vi "correction_data.vi"() -> ()   [LabVIEW 2020]
uses:
  CasaoManagerGeneralSpecifications.ctl
  General dimensions definition.ctl
  Point2D.ctl
  Point2Df.ctl
  WavefrontCorrector.lvclass
  Camera.lvclass
  CorrectionDataManager.lvclass
  Image.lvclass
  HasoEngine.lvclass
  InteractionMatrixAcquisitionParameters.ctl
  HasoSlopes.lvclass
  Data alignment enum.ctl
  InteractionMatrixToCommandMatrixParameters.ctl
panel:
  out "Camera Image (2N)":u32[][](graph)
  in  "Start Acq":bool
  out "Camera Image (2N+1)":u32[][](graph)
  in  "number of images to sum":u32=1
  in  "Exposure time (us)":i32=1000
  out "# of valid actuators":u32
  out "Singular values":dbl[](graph)
  in  "Correction data file name":string="Data\\data_correction_manager_example.aomi"
  in  "WavefrontCorrector Configuration file path":path
  out "error out":errorcluster
  out "Informations extracted \nfrom configuration files":T1 caption="Informations extracted from configuration files"
  in  "Haso configuration file path":path
  # "This example is Hardware-dependant, \nplease use your own Haso and corrector configuration file and acquisition system"
  # "Acquisition parameters"
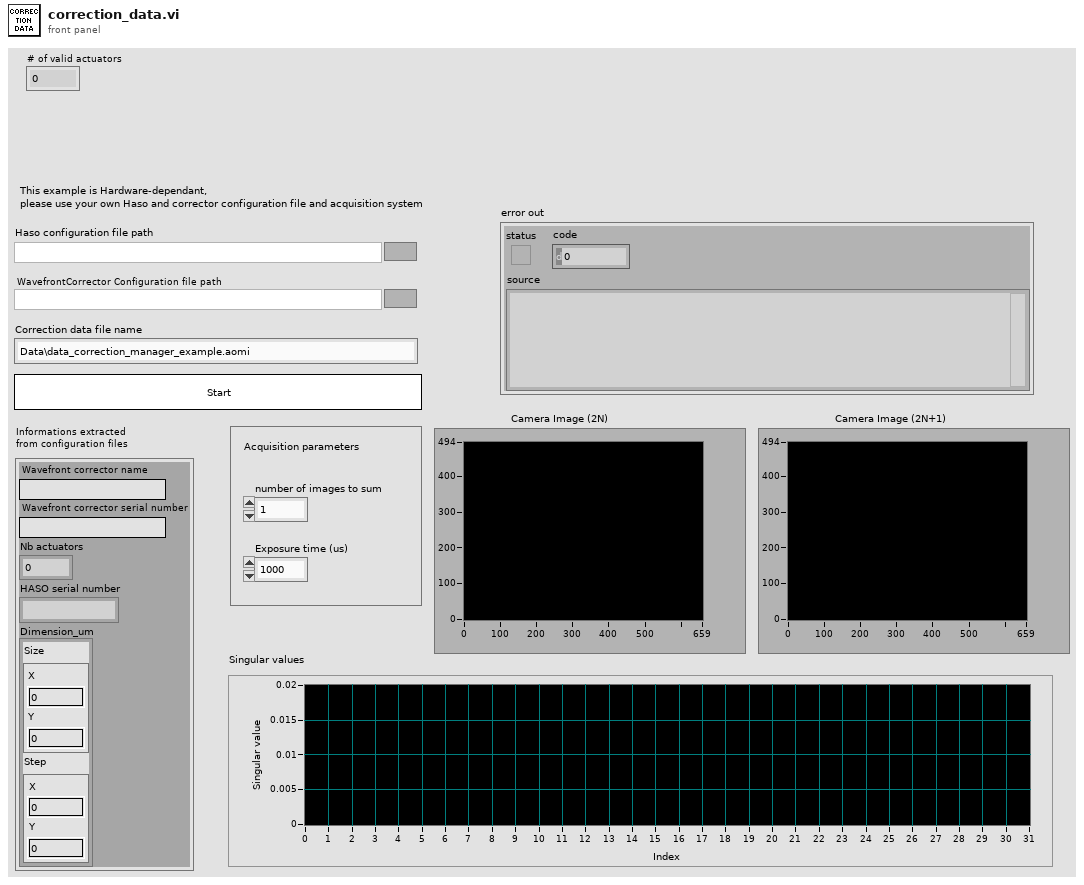
[diagram p1: front panel]
types:
  T1 = typedef "CasaoManagerGeneralSpecifications.ctl" = cluster{"Wavefront corrector name":string, "Wavefront corrector serial number":string, "Nb actuators":i32, "HASO serial number":string, "Dimension_um":T2}
  T2 = typedef "General dimensions definition.ctl" = cluster{"Size":T3, "Step":T4}
  T3 = typedef "Point2D.ctl" = cluster{"X":u32, "Y":u32}
  T4 = typedef "Point2Df.ctl" = cluster{"X":sgl, "Y":sgl}
  T5 = typedef "InteractionMatrixAcquisitionParameters.ctl" = cluster{"Push - Pull value":sgl}
  T6 = typedef "Data alignment enum.ctl" = enum16{"8", "16", "32"}
  T7 = typedef "InteractionMatrixToCommandMatrixParameters.ctl" = cluster{"Number of kept modes":i32, "Tilt filtering":bool}
  T8 = typedef "Wavefront Corrector states - ONE.ctl" = cluster{"Max":sgl, "Min":sgl, "Validity":enum16{"valid", "fixed", "invalid"}, "Fixed_Position":sgl}
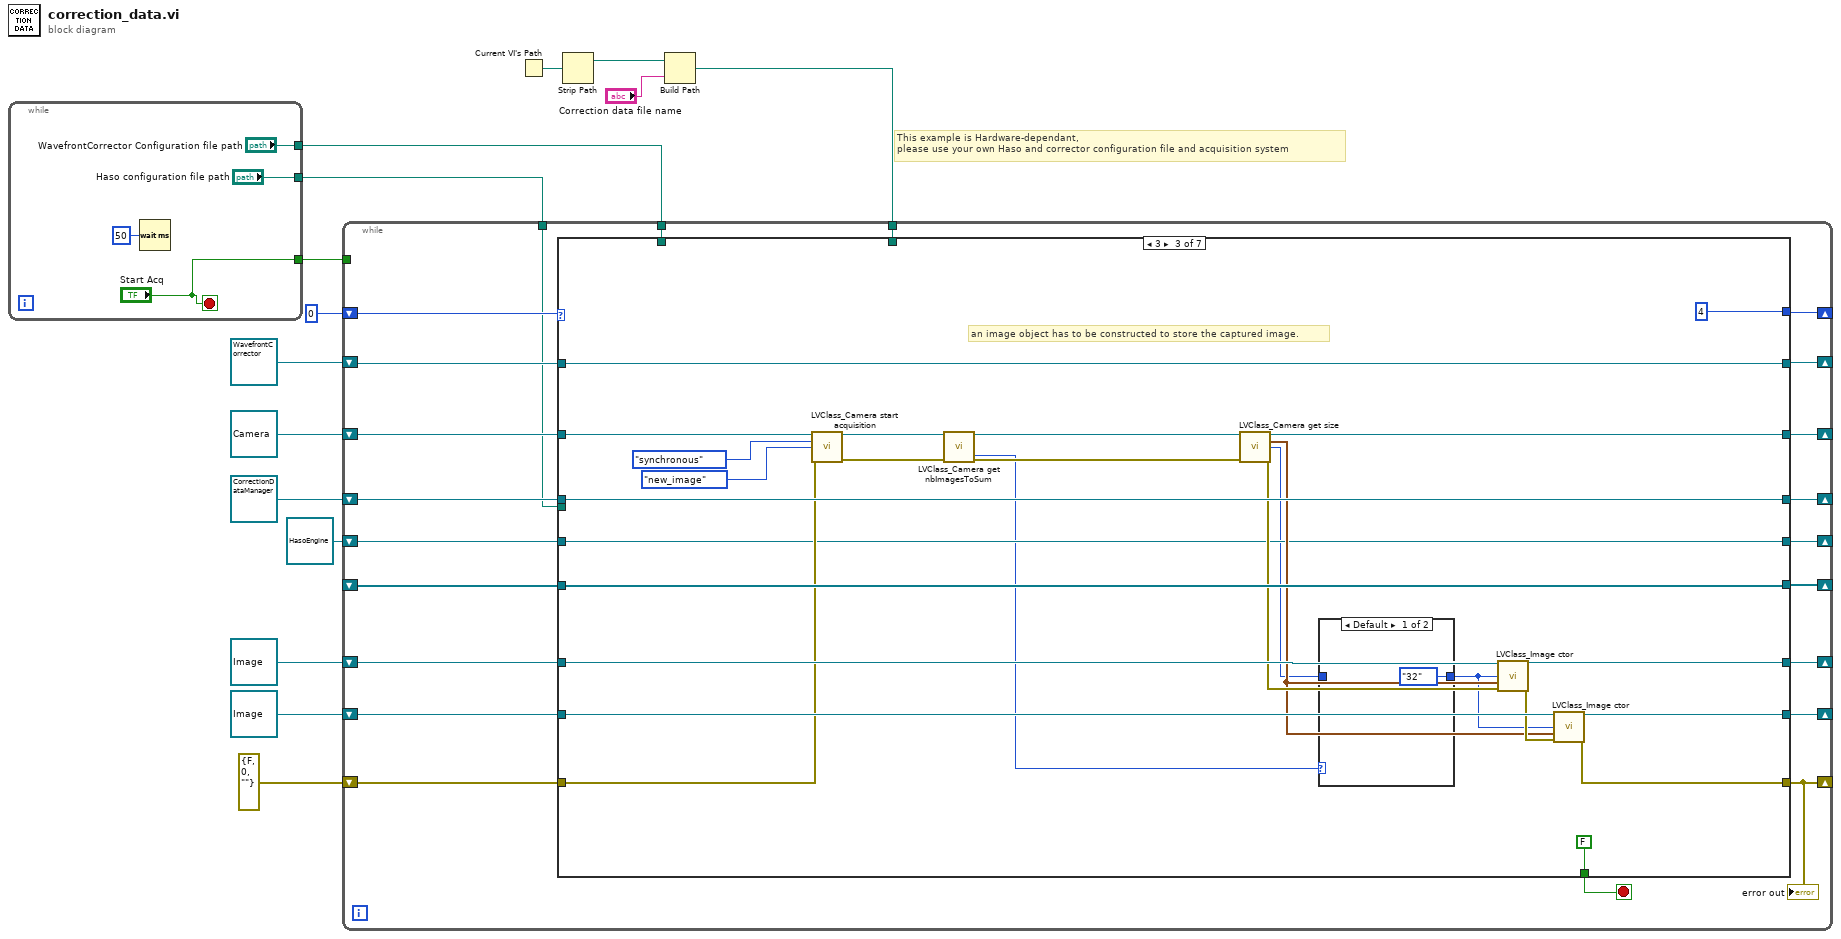
[diagram p0: block diagram]
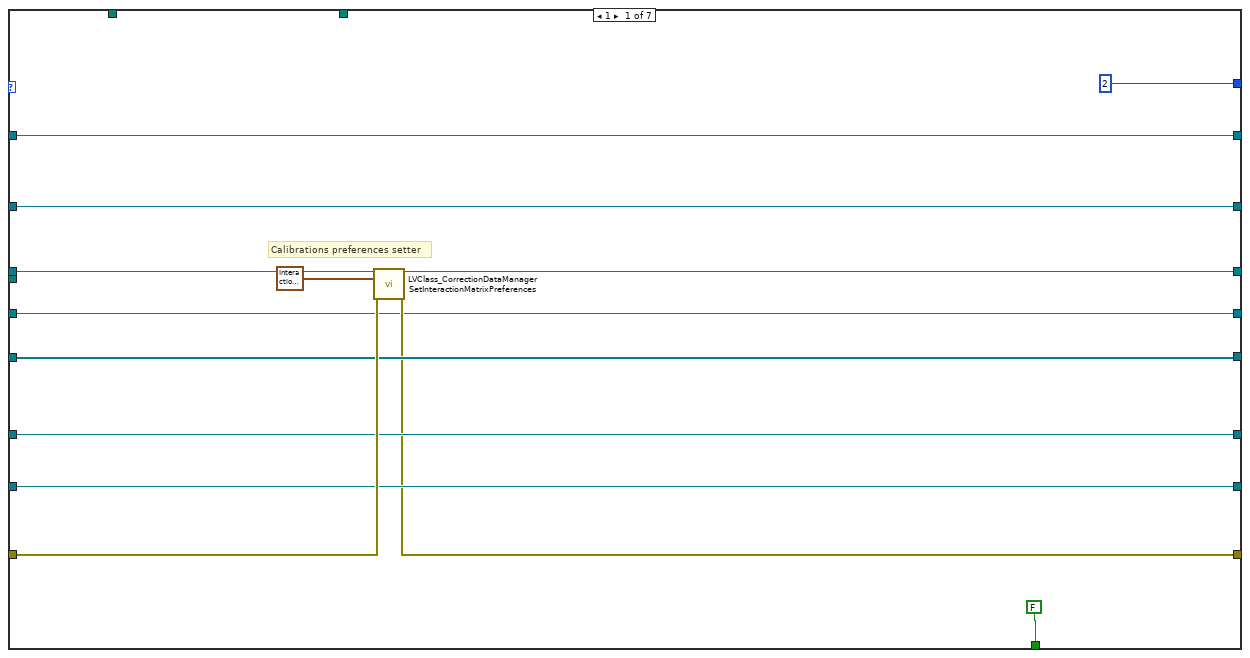
[diagram p2: hidden frame]
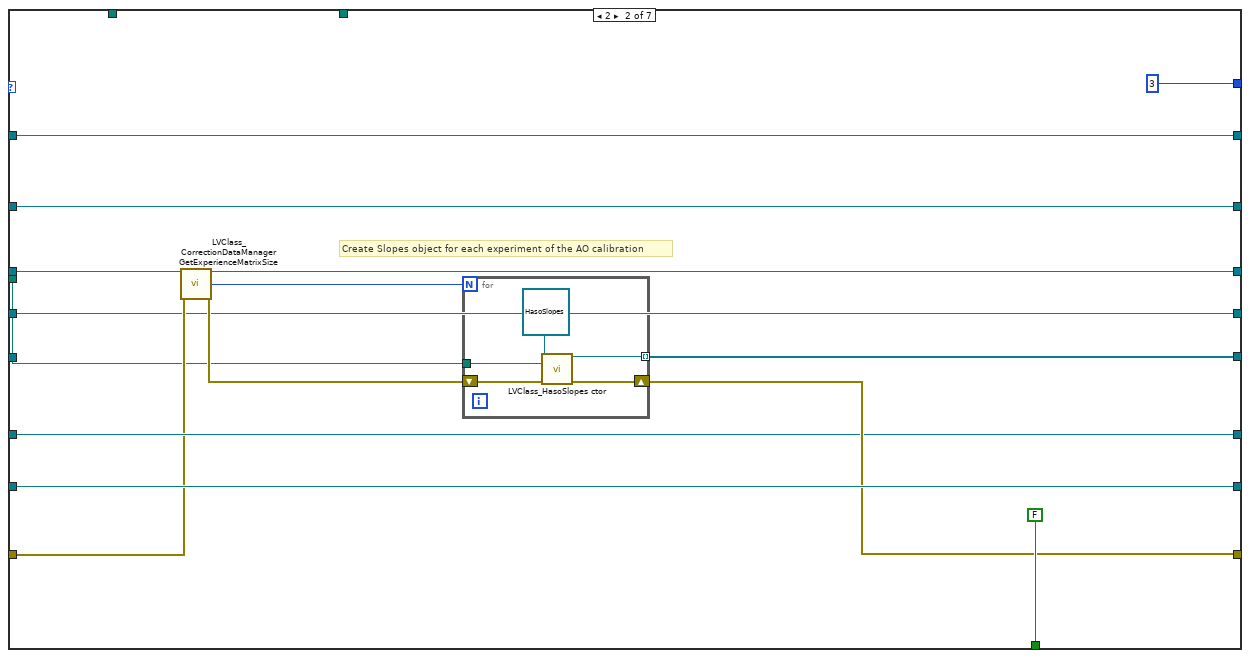
[diagram p3: hidden frame]
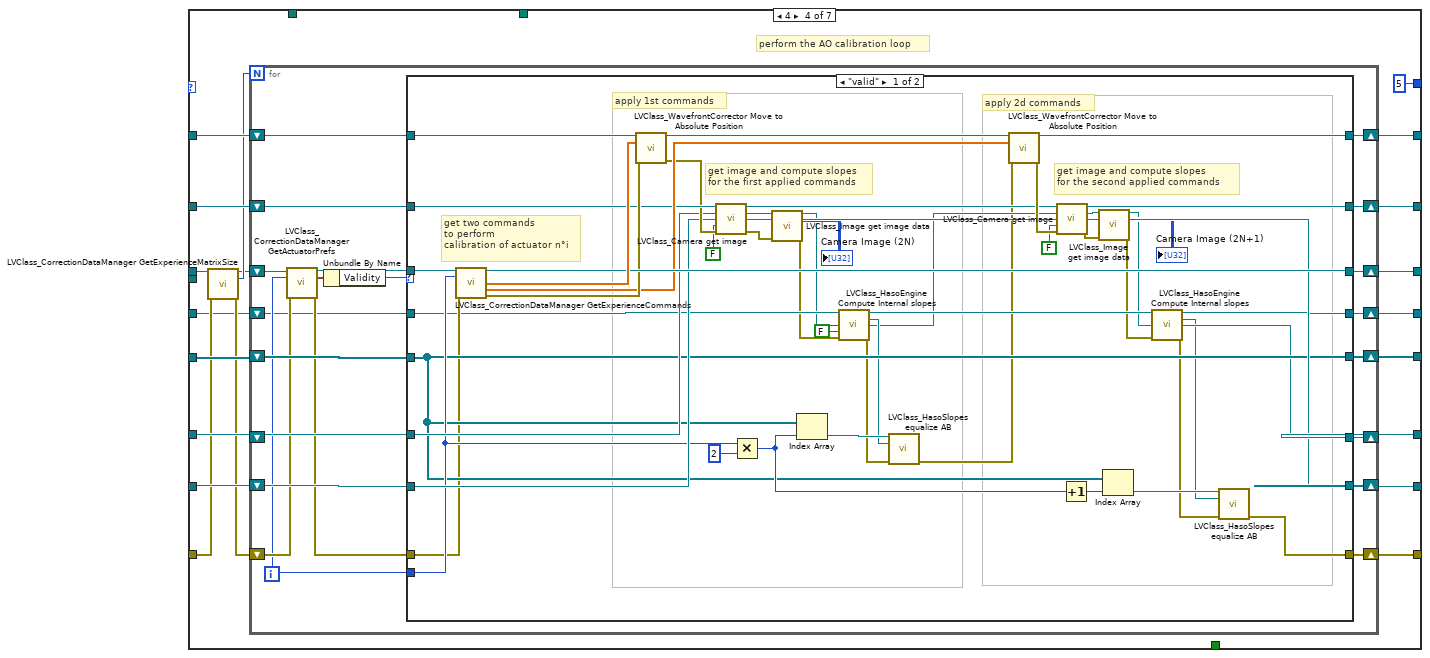
[diagram p5: hidden frame]
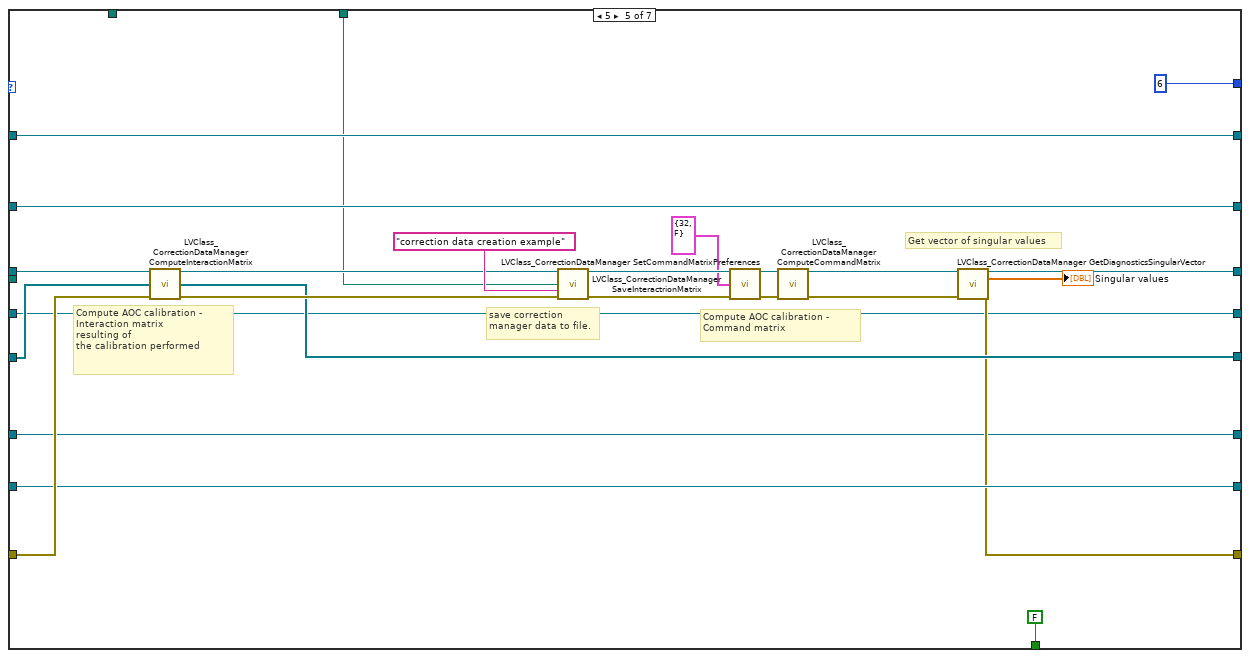
[diagram p7: hidden frame]
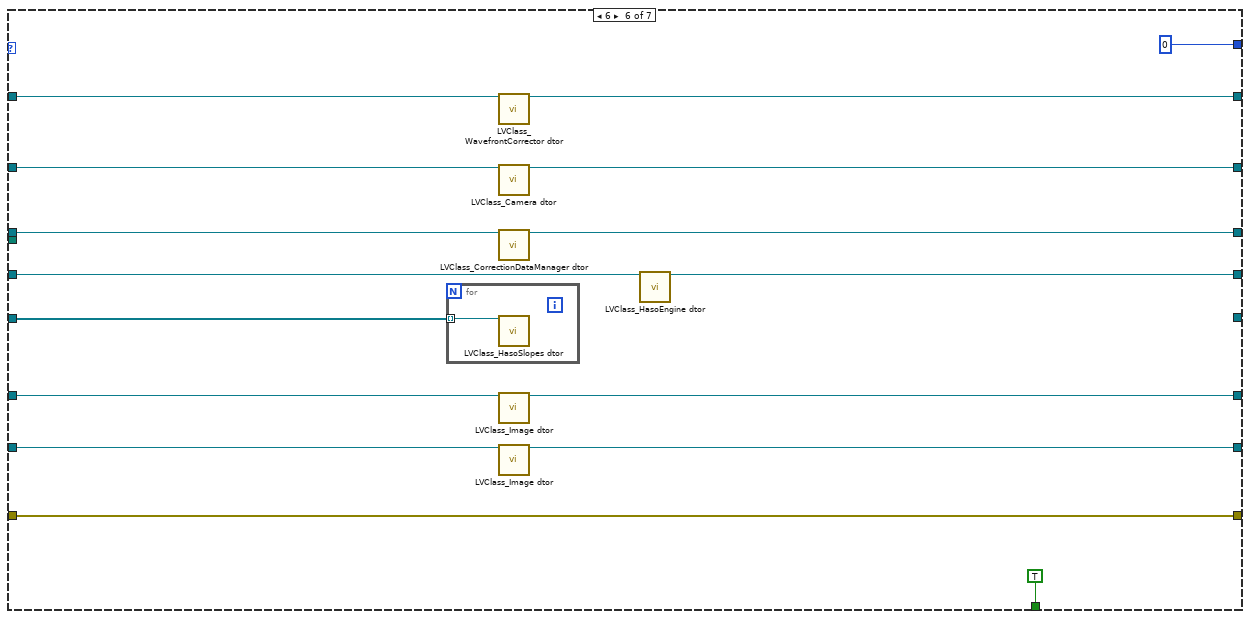
[diagram p8: hidden frame]
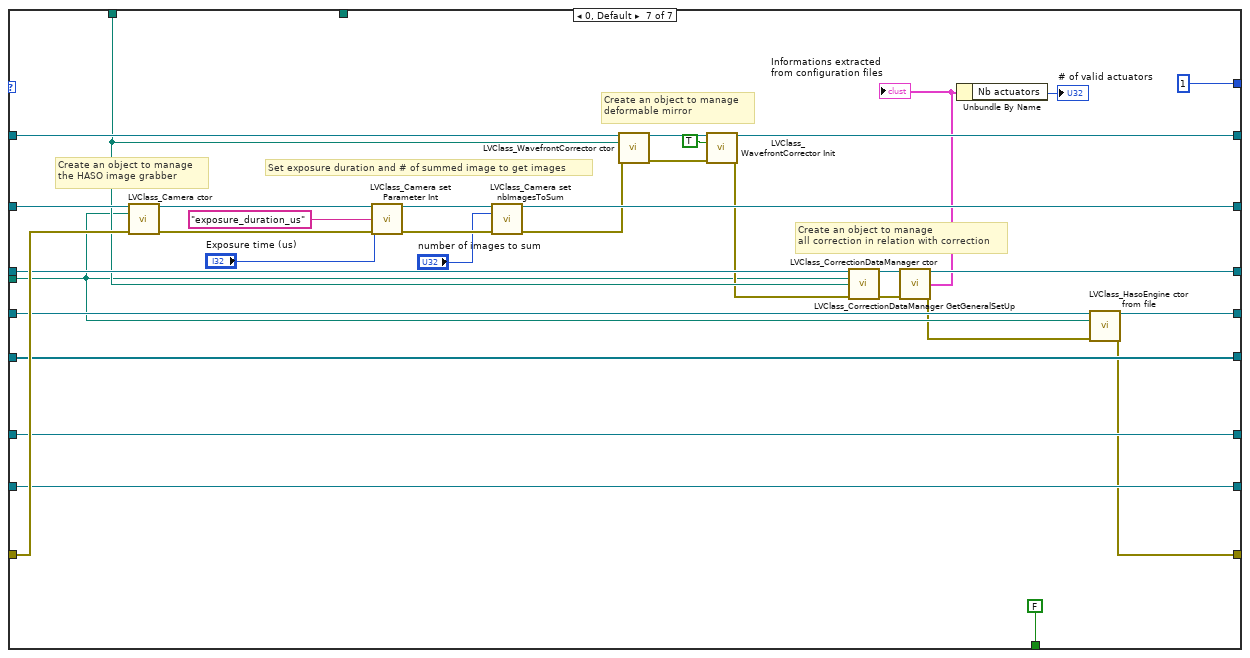
[diagram p9: hidden frame]
diagram:
  # "This example is Hardware-dependant, \nplease use your own Haso and corrector configuration file and acquisition system"
  n1 = while {
    tunnel: ["Start Acq"] -> w9
    tunnel: ["Haso configuration file path"] -> w2
    tunnel: ["WavefrontCorrector Configuration file path"] -> w1
    stop <- "Start Acq" stop-if-true
    n2 = Wait (ms)(milliseconds to wait=u32 50) -> ()  [unwired: 1 out]
  }
  n3 = Current VI's Path() -> (path=w6:path)
  n4 = Strip Path(path=w6) -> (stripped path=w8:path)  [unwired: 1 out]
  n5 = Build Path(base path=w8, name or relative path="Correction data file name") -> (appended path=w5:path)
  n6 = while {
    shift-right: [w33] -> _
    shift-left: refnum<class "WavefrontCorrector.lvclass"> refnum ("WavefrontCorrector in") -> [w35]
    shift-right: [w31] -> _
    shift-left: refnum<class "Camera.lvclass"> refnum ("Camera") -> [w38]
    shift-right: [w32] -> _
    shift-left: refnum<class "CorrectionDataManager.lvclass"> refnum ("CorrectionDataManager in") -> [w34]
    shift-right: [w28] -> _
    shift-left: refnum<class "Image.lvclass"> refnum ("Image in") -> [w30]
    shift-right: [w40] -> _
    shift-left: 0 -> [w41]
    shift-right: [w26] -> _
    shift-left: errorcluster {"status"=FALSE, "code"=0, "source"=""} ("error out") -> [w37]
    tunnel: w1 -> [w36]
    tunnel: w2 -> [w22]
    shift-right: [w29] -> _
    shift-left: _ -> [w27]
    shift-right: [w24] -> _
    shift-left: refnum<class "Image.lvclass"> refnum ("Image out") -> [w25]
    tunnel: w9 -> [_]
    tunnel: w5 -> [w23]
    shift-right: [w20] -> _
    shift-left: refnum<class "HasoEngine.lvclass"> refnum ("HasoEngine out") -> [w21]
    stop <- w39 stop-if-true
    n7 = case shown="3" w41 {
      tunnel: [2 3 4 5 6 0 1] -> w40
      tunnel: [FALSE FALSE FALSE _ FALSE TRUE FALSE] -> w39
      tunnel: w38 -> [w47 w65 w83 w115 w206 w239 w274]
      tunnel: [w43 w63 w96 w116 w204 w229 w244] -> w26
      tunnel: w37 -> [w50 w60 w84 w106 w221 w229 w273]
      tunnel: w36 -> [_ _ _ _ _ _ w270]
      tunnel: w35 -> [w48 w66 w94 w121 w207 w238 w272]
      tunnel: w22 -> [_ w56 _ _ _ _ w246]
      tunnel: w34 -> [w51 w58 w93 w109 w223 w235 w271]
      tunnel: [w48 w66 w94 w118 w207 w234 w264] -> w33
      tunnel: [w44 w57 w93 w117 w208 w228 w251] -> w32
      tunnel: [w47 w65 w95 w114 w206 w233 w261] -> w31
      tunnel: w30 -> [w46 w64 w98 w113 w205 w236 w268]
      tunnel: [w49 w67 w92 w119 w210 _ w269] -> w29
      tunnel: [w46 w64 w97 w110 w205 w232 w268] -> w28
      tunnel: w27 -> [w49 _ w92 w120 w222 w237 w269]
      tunnel: w25 -> [w45 w62 w91 w112 w203 w231 w267]
      tunnel: [w45 w62 w90 w111 w203 w230 w267] -> w24
      tunnel: w23 -> [_ _ _ _ w202 _ _]
      tunnel: w21 -> [w42 w55 w82 w104 w201 w227 w247]
      tunnel: [w42 w55 w82 w103 w201 w226 w243] -> w20
      frame 1 {
        # "Calibrations preferences setter"
        n8 = call "LVClass_CorrectionDataManager SetInteractionMatrixPreferences.vi"("CorrectionDataManager in"=w51, "push_pull_value"=T5 {"Push - Pull value"=0.2} ("Interaction Matrix Parameters 2"), "error in (no error)"=w50) -> ("CorrectionDataManager out"=w44:refnum<class "CorrectionDataManager.lvclass">, "error out"=w43:errorcluster)  [unwired: 11 in]
      }
      frame 2 {
        # "Create Slopes object for each experiment of the AO calibration"
        n9 = call "LVClass_CorrectionDataManager GetExperienceMatrixSize.vi"("CorrectionDataManager in"=w58, "error in (no error)"=w60) -> ("CorrectionDataManager out"=w57:refnum<class "CorrectionDataManager.lvclass">, "# of experiments"=w61:u32, "error out"=w59:errorcluster)  [unwired: 10 in, 1 out]
        n10 = for {
          N: w61 -> [_]
          tunnel: w56 -> [w74]
          tunnel: [w72] -> w67 mode=indexing
          shift-right: [w71] -> w63
          shift-left: w59 -> [w70]
          n11 = call "LVClass_HasoSlopes ctor.vi"("HasoSlopes in"=refnum<class "HasoSlopes.lvclass"> refnum, "Configuration file path"=w74, "error in (no error)"=w70) -> ("HasoSlopes out"=w72:refnum<class "HasoSlopes.lvclass">, "error out"=w71:errorcluster)  [unwired: 11 in]
        }
      }
      frame 3 {
        # "an image object has to be constructed to store the captured image."
        n12 = call "LVClass_Camera start acquisition.vi"("Camera in"=w83, "synchronisation_mode"=enum16{"synchronous", "asynchronous"}."synchronous", "acquisition_mode"=enum16{"last_image", "new_image"}."new_image", "error in (no error)"=w84) -> ("Camera out"=w81:refnum<class "Camera.lvclass">, "error out"=w80:errorcluster)  [unwired: 10 in]
        n13 = call "LVClass_Camera get nbImagesToSum.vi"("Camera in"=w81, "error in (no error)"=w80) -> ("Camera out"=w78:refnum<class "Camera.lvclass">, "nb_image"=w77:u32, "error out"=w79:errorcluster)  [unwired: 11 in]
        n14 = call "LVClass_Camera get size.vi"("Camera in"=w78, "error in (no error)"=w79) -> ("Camera out"=w95:refnum<class "Camera.lvclass">, "size"=w87:T3, "Number of bits"=w75:T6, "error out"=w89:errorcluster)  [unwired: 10 in]
        n15 = case shown="Default" w77 {
          tunnel: [Data_alignment_enum."32" ("Number of bits") w102] -> w76
          tunnel: w75 -> [_ w102]
          frame Default {
          }
          frame 1 {
          }
        }
        n16 = call "LVClass_Image ctor.vi"("Image in"=w91, "Data alignment"=w76, "Size"=w87, "error in (no error)"=w89) -> ("Image out"=w90:refnum<class "Image.lvclass">, "error out"=w88:errorcluster)  [unwired: 10 in]
        n17 = call "LVClass_Image ctor.vi"("Image in"=w98, "Data alignment"=w76, "Size"=w87, "error in (no error)"=w88) -> ("Image out"=w97:refnum<class "Image.lvclass">, "error out"=w96:errorcluster)  [unwired: 10 in]
      }
      frame 4 {
        # "perform the AO calibration loop"
        n18 = call "LVClass_CorrectionDataManager GetExperienceMatrixSize.vi"("CorrectionDataManager in"=w109, "error in (no error)"=w106) -> ("CorrectionDataManager out"=w107:refnum<class "CorrectionDataManager.lvclass">, "# of valid actuators"=w108:u32, "error out"=w105:errorcluster)  [unwired: 10 in, 1 out]
        n19 = for {
          N: w108 -> [_]
          shift-right: [w142] -> w117
          shift-left: w107 -> [w141]
          shift-right: [w137] -> w118
          shift-left: w121 -> [w143]
          shift-right: [w136] -> w116
          shift-left: w105 -> [w129]
          shift-right: [w134] -> w114
          shift-left: w115 -> [w135]
          shift-right: [w131] -> w111
          shift-left: w112 -> [w132]
          shift-right: [w130] -> w110
          shift-left: w113 -> [w133]
          shift-right: [w138] -> w119
          shift-left: w120 -> [w139]
          shift-right: [w123] -> w103
          shift-left: w104 -> [w124]
          i -> [w125]
          n20 = call "LVClass_CorrectionDataManager GetActuatorPrefs.vi"("CorrectionDataManager in"=w141, "N° actuator"=w125, "error in (no error)"=w129) -> ("CorrectionDataManager out"=w140:refnum<class "CorrectionDataManager.lvclass">, "Actuator state"=w128:T8, "error out"=w127:errorcluster)  [unwired: 10 in]
          n21 = Unbundle By Name(w128) -> ("Validity"=w126:enum16{"valid", "fixed", "invalid"})
          n22 = case shown="\"valid\"" w126 {
            tunnel: w143 -> [w192 w200]
            tunnel: [w190 w195] -> w142
            tunnel: w140 -> [w189 w195]
            tunnel: w139 -> [w163 w196]
            tunnel: [w163 w196] -> w138
            tunnel: [w185 w200] -> w137
            tunnel: [w144 w194] -> w136
            tunnel: w135 -> [w184 w199]
            tunnel: [w180 w199] -> w134
            tunnel: w133 -> [w178 w197]
            tunnel: w132 -> [w179 w198]
            tunnel: [w150 w198] -> w131
            tunnel: [w174 w197] -> w130
            tunnel: w127 -> [w160 w194]
            tunnel: w125 -> [w164 _]
            tunnel: w124 -> [w159 w193]
            tunnel: [w153 w193] -> w123
            frame "valid" {
              # "apply 2d commands"
              # "apply 1st commands"
              # "get image and compute slopes\nfor the second applied commands"
              # "get image and compute slopes\nfor the first applied commands"
              # "get two commands\nto perform \ncalibration of actuator n°i"
              n23 = call "LVClass_CorrectionDataManager GetExperienceCommands.vi"("CorrectionDataManager in"=w189, "N° actuator"=w164, "error in (no error)"=w160) -> ("CorrectionDataManager out"=w190:refnum<class "CorrectionDataManager.lvclass">, "First DeltaCommand"=w191:sgl[], "Second DeltaCommand"=w186:sgl[], "error out"=w188:errorcluster)  [unwired: 9 in]
              n24 = call "LVClass_WavefrontCorrector Move to Absolute Position.vi"("WavefrontCorrector in"=w192, "Absolute Positions"=w191, "error in (no error)"=w188) -> ("WavefrontCorrector out"=w187:refnum<class "WavefrontCorrector.lvclass">, "error out"=w183:errorcluster)  [unwired: 11 in]
              n25 = call "LVClass_Camera get image.vi"("Camera in"=w184, "Image"=w179, "Image RAW"=w178, "remove_background"=FALSE, "error in (no error)"=w183) -> ("Camera out"=w181:refnum<class "Camera.lvclass">, "Image (dup)"=w166:refnum<class "Image.lvclass">, "Image (dup) RAW"=w176:refnum<class "Image.lvclass">, "error out"=w165:errorcluster)  [unwired: 7 in]
              n26 = Multiply(x=w164, y=2) -> (x*y=w171:i32)
              n27 = call "LVClass_Image get image data.vi"("Image in"=w166, "error in (no error)"=w165) -> ("Image out"=w156:refnum<class "Image.lvclass">, "Image data out"=→"Camera Image (2N)":u32[][], "error out"=w154:errorcluster)  [unwired: 11 in]
              n28 = Index Array(array=w163, index=w171) -> (element=w170:refnum<class "HasoSlopes.lvclass">)
              n29 = call "LVClass_HasoEngine Compute Internal slopes.vi"("HasoEngine in"=w159, "Image.lvclass"=w156, "learn_from_trimmer"=FALSE, "error in (no error)"=w154) -> ("HasoEngine out"=w158:refnum<class "HasoEngine.lvclass">, "HasoSlopes (dup)"=w157:refnum<class "HasoSlopes.lvclass">, "Image (dup)"=w146:refnum<class "Image.lvclass">, "error out"=w152:errorcluster)  [unwired: 7 in, 1 out]
              n30 = call "LVClass_HasoSlopes equalize AB.vi"("HasoSlopes dest in"=w170, "HasoSlopes source in"=w157, "error in (no error)"=w152) -> ("error out"=w145:errorcluster)  [unwired: 10 in, 2 out]
              n31 = call "LVClass_WavefrontCorrector Move to Absolute Position.vi"("WavefrontCorrector in"=w187, "Absolute Positions"=w186, "error in (no error)"=w145) -> ("WavefrontCorrector out"=w185:refnum<class "WavefrontCorrector.lvclass">, "error out"=w182:errorcluster)  [unwired: 11 in]
              n32 = call "LVClass_Camera get image.vi"("Camera in"=w181, "Image"=w146, "Image RAW"=w176, "remove_background"=FALSE, "error in (no error)"=w182) -> ("Camera out"=w180:refnum<class "Camera.lvclass">, "Image (dup)"=w162:refnum<class "Image.lvclass">, "Image (dup) RAW"=w174:refnum<class "Image.lvclass">, "error out"=w161:errorcluster)  [unwired: 7 in]
              n33 = Increment(x=w171) -> (x+1=w169:i32)
              n34 = call "LVClass_Image get image data.vi"("Image in"=w162, "error in (no error)"=w161) -> ("Image out"=w151:refnum<class "Image.lvclass">, "Image data out"=→"Camera Image (2N+1)":u32[][], "error out"=w149:errorcluster)  [unwired: 11 in]
              n35 = Index Array(array=w163, index=w169) -> (element=w168:refnum<class "HasoSlopes.lvclass">)
              n36 = call "LVClass_HasoEngine Compute Internal slopes.vi"("HasoEngine in"=w158, "Image.lvclass"=w151, "error in (no error)"=w149) -> ("HasoEngine out"=w153:refnum<class "HasoEngine.lvclass">, "HasoSlopes (dup)"=w147:refnum<class "HasoSlopes.lvclass">, "Image (dup)"=w150:refnum<class "Image.lvclass">, "error out"=w148:errorcluster)  [unwired: 8 in, 1 out]
              n37 = call "LVClass_HasoSlopes equalize AB.vi"("HasoSlopes dest in"=w168, "HasoSlopes source in"=w147, "error in (no error)"=w148) -> ("error out"=w144:errorcluster)  [unwired: 10 in, 2 out]
            }
            frame "fixed", Default {
            }
          }
        }
      }
      frame 5 {
        # "Compute AOC calibration - Interaction matrix\nresulting of\nthe calibration performed"
        # "Compute AOC calibration - Command matrix"
        # "Get vector of singular values"
        # "save correction\nmanager data to file."
        n38 = call "LVClass_CorrectionDataManager ComputeInteractionMatrix.vi"("CorrectionDataManager in"=w223, "HasoSlopes array"=w222, "error in (no error)"=w221) -> ("CorrectionDataManager out"=w212:refnum<class "CorrectionDataManager.lvclass">, "HasoSlopes array 2"=w210:refnum<class "HasoSlopes.lvclass">[], "error out"=w211:errorcluster)  [unwired: 10 in]
        n39 = call "LVClass_CorrectionDataManager SaveInteractrionMatrix.vi"("CorrectionDataManager in"=w212, "Interaction Matrix file path"=w202, "comment"="correction data creation example", "error in (no error)"=w211) -> ("CorrectionDataManager out"=w216:refnum<class "CorrectionDataManager.lvclass">, "error out"=w213:errorcluster)  [unwired: 10 in]
        n40 = call "LVClass_CorrectionDataManager SetCommandMatrixPreferences.vi"("CorrectionDataManager in"=w216, "Prefs"=T7 {"Number of kept modes"=32, "Tilt filtering"=FALSE}, "error in (no error)"=w213) -> ("CorrectionDataManager out"=w217:refnum<class "CorrectionDataManager.lvclass">, "error out"=w220:errorcluster)  [unwired: 11 in]
        n41 = call "LVClass_CorrectionDataManager ComputeCommandMatrix.vi"("CorrectionDataManager in"=w217, "error in (no error)"=w220) -> ("CorrectionDataManager out"=w218:refnum<class "CorrectionDataManager.lvclass">, "error out"=w219:errorcluster)  [unwired: 12 in]
        n42 = call "LVClass_CorrectionDataManager GetDiagnosticsSingularVector.vi"("CorrectionDataManager in"=w218, "error in (no error)"=w219) -> ("CorrectionDataManager out"=w208:refnum<class "CorrectionDataManager.lvclass">, "ArrayOfSingularValues"=→"Singular values":dbl[], "error out"=w204:errorcluster)  [unwired: 11 in]
      }
      frame 6 {
        n43 = for {
          tunnel: w237 -> [w242] mode=indexing
          n44 = call "LVClass_HasoSlopes dtor.vi"("HasoSlopes in"=w242) -> ()  [unwired: 13 in, 2 out]
        }
        n45 = call "LVClass_WavefrontCorrector dtor.vi"("WavefrontCorrector in"=w238) -> ("WavefrontCorrector out"=w234:refnum<class "WavefrontCorrector.lvclass">)  [unwired: 13 in, 1 out]
        n46 = call "LVClass_Camera dtor.vi"("Camera in"=w239) -> ("Camera out"=w233:refnum<class "Camera.lvclass">)  [unwired: 13 in, 1 out]
        n47 = call "LVClass_CorrectionDataManager dtor.vi"("CorrectionDataManager in"=w235) -> ("CorrectionDataManager out"=w228:refnum<class "CorrectionDataManager.lvclass">)  [unwired: 13 in, 1 out]
        n48 = call "LVClass_Image dtor.vi"("Image in"=w231) -> ("Image out"=w230:refnum<class "Image.lvclass">)  [unwired: 13 in, 1 out]
        n49 = call "LVClass_Image dtor.vi"("Image in"=w236) -> ("Image out"=w232:refnum<class "Image.lvclass">)  [unwired: 13 in, 1 out]
        n50 = call "LVClass_HasoEngine dtor.vi"("HasoEngine in"=w227) -> ("HasoEngine out"=w226:refnum<class "HasoEngine.lvclass">)  [unwired: 13 in, 1 out]
      }
      frame 0, Default {
        # "Create an object to manage \nall correction in relation with correction"
        # "Set exposure duration and # of summed image to get images"
        # "Create an object to manage \ndeformable mirror"
        # "Create an object to manage \nthe HASO image grabber"
        n51 = call "LVClass_Camera ctor.vi"("Camera"=w274, "Configuration file path"=w246, "error in (no error)"=w273) -> ("Camera (new)"=w256:refnum<class "Camera.lvclass">, "error out"=w255:errorcluster)  [unwired: 11 in]
        n52 = call "LVClass_Camera set Parameter Int.vi"("Camera in"=w256, "parameter_name"="exposure_duration_us", "value"="Exposure time (us)", "error in (no error)"=w255) -> ("Camera out"=w262:refnum<class "Camera.lvclass">, "error out"=w260:errorcluster)  [unwired: 10 in]
        n53 = call "LVClass_Camera set nbImagesToSum.vi"("Camera in"=w262, "nb_image"="number of images to sum", "error in (no error)"=w260) -> ("Camera out"=w261:refnum<class "Camera.lvclass">, "error out"=w254:errorcluster)  [unwired: 11 in]
        n54 = call "LVClass_WavefrontCorrector ctor.vi"("WavefrontCorrector in"=w272, "PathToWavefrontCorrectorSetupFile"=w270, "error in (no error)"=w254) -> ("WavefrontCorrector out"=w265:refnum<class "WavefrontCorrector.lvclass">, "error out"=w263:errorcluster)  [unwired: 11 in]
        n55 = call "LVClass_WavefrontCorrector Init.vi"("WavefrontCorrector in"=w265, "set_init_state_from_config_file"=TRUE, "error in (no error)"=w263) -> ("WavefrontCorrector out"=w264:refnum<class "WavefrontCorrector.lvclass">, "error out"=w253:errorcluster)  [unwired: 11 in]
        n56 = call "LVClass_CorrectionDataManager ctor.vi"("CorrectionDataManager in"=w271, "PathTohaso_config_file_path"=w246, "PathTowfc_config_file_path"=w270, "error in (no error)"=w253) -> ("CorrectionDataManager out"=w252:refnum<class "CorrectionDataManager.lvclass">, "error out"=w250:errorcluster)  [unwired: 10 in]
        n57 = call "LVClass_CorrectionDataManager GetGeneralSetUp.vi"("CorrectionDataManager in"=w252, "error in (no error)"=w250) -> ("CorrectionDataManager out"=w251:refnum<class "CorrectionDataManager.lvclass">, "general"=w248:T1, "error out"=w245:errorcluster)  [unwired: 11 in]
        "Informations extracted \nfrom configuration files" <- w248
        n58 = Unbundle By Name(w248) -> ("Nb actuators"=→"# of valid actuators":i32)
        n59 = call "LVClass_HasoEngine ctor from file.vi"("HasoEngine in"=w247, "Configuration file path"=w246, "error in (no error)"=w245) -> ("HasoEngine out"=w243:refnum<class "HasoEngine.lvclass">, "error out"=w244:errorcluster)  [unwired: 11 in]
      }
    }
    "error out" <- w26
  }
